vi "PoseAndTargeting.vi"() -> ()   [LabVIEW 2020]
doc: "Manages the robot's pose (position, heading, and velocity) and targeting information. Data from the IMU, swerve drive encoders, swerve azimuth encoders, turret enoder, and LimeLight are fused together to estimate these values. Supports pose resets on boot, from the Autonomous Sequencer, and on command from the FRC 4265 Dashboard."
uses:
  c71665c3-219d-469c-9b81-2f0818bb1921.vi
  sensordata.vi
  driverdata.vi
  robotoutputs.vi
panel:
  in  "Firing Delay (s)":dbl
  in  "Radial Target Shift (in)":dbl
  in  "Angular Target Shift (deg)":dbl
  in  "Min Timed Aligned (ms)":u32=500
  in  "Acceptable Heading Error (deg)":dbl=4.0
  in  "Vision Trust Threshold (in)":dbl=10.0
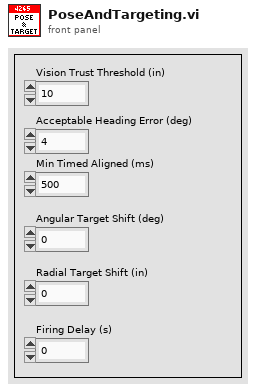
[diagram p1: front panel]
types:
  T1 = enum16{"Normal", "Auto Set", "Reset IMU", "Manual Push", "Init"}
  T2 = enum16{"Center", "North", "NorthWest", "West", "SouthWest", "South", "SouthEast", "East", "NorthEast"}
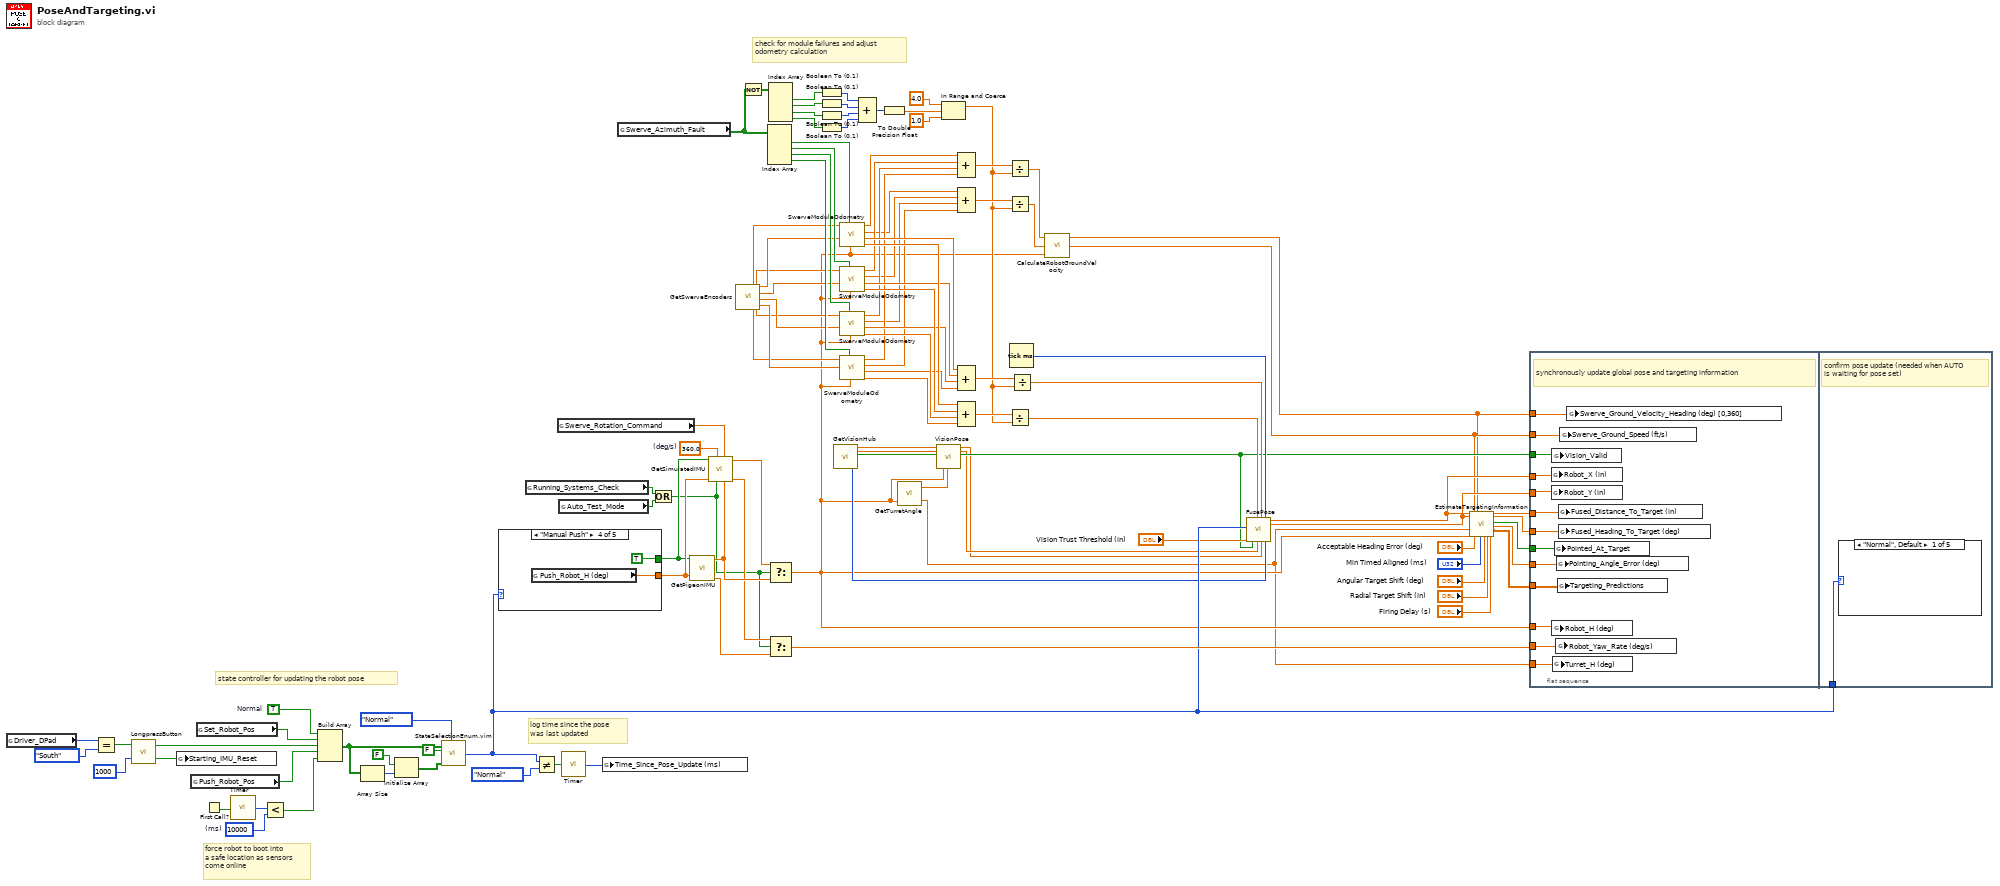
[diagram p0: block diagram]
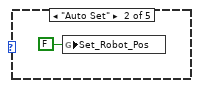
[diagram p2: hidden frame]
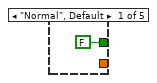
[diagram p6: hidden frame]
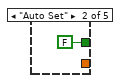
[diagram p7: hidden frame]
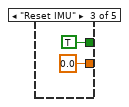
[diagram p8: hidden frame]
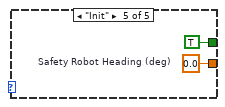
[diagram p9: hidden frame]
diagram:
  w79 = 360.0  # (deg/s)
  w83 = u32 10000  # (ms)
  w89 = TRUE  # Normal
  # "force robot to boot into\na safe location as sensors\ncome online"
  # "log time since the pose\nwas last updated"
  # "state controller for updating the robot pose"
  # "check for module failures and adjust\nodometry calculation"
  n1 = global read "driverdata.vi" "Driver_DPad"() -> (w46:T2)
  n2 = Equal?(x=w46, y=T2."South") -> (x = y?=w45:bool)
  n3 = call "LongpressButton.vi"("Threshold (ms)"=u32 1000, "Button"=w45) -> ("Starting Press"=w42:bool, "Longpress Button"=w43:bool)
  n4 = global write "driverdata.vi" "Starting_IMU_Reset"(w42) -> ()
  n5 = global read "sensordata.vi" "Push_Robot_Pos"() -> (w90:bool)
  n6 = global read "sensordata.vi" "Set_Robot_Pos"() -> (w78:bool)
  n7 = First Call?() -> (First Call?: T/F=w86:bool)
  n8 = call "Timer.vi"("Reset Timer"=w86) -> ("Time (ms)"=w85:u32)
  n9 = Less?(x=w85, y=w83) -> (x < y?=w84:bool)
  n10 = Build Array(w89, w78, w43, w90, w84) -> (w38:bool[])
  n11 = Array Size(array=w38) -> (size(s)=w41:i32)
  n12 = Initialize Array(FALSE, w41) -> (w37:bool[])
  n13 = call "StateSelectionEnum.vim"("Enum Def"=T1."Normal", "Disallowed States"=w37, "Enable Edge Trigger"=FALSE, "State Triggers"=w38) -> ("Selected State"=w28:T1)  [unwired: 1 in, 1 out]
  n14 = case shown="\"Manual Push\"" w28 {
    tunnel: [_ _ 0.0 ("Push_Robot_H (deg)") w118 w119] -> w82
    tunnel: [FALSE FALSE TRUE TRUE TRUE] -> w81
    frame "Normal", Default {
    }
    frame "Auto Set" {
    }
    frame "Reset IMU" {
    }
    frame "Manual Push" {
      n15 = global read "sensordata.vi" "Push_Robot_H (deg)"() -> (w118:dbl)
    }
    frame "Init" {
      w119 = 0.0  # Safety Robot Heading (deg)
    }
  }
  n16 = global read "driverdata.vi" "Running_Systems_Check"() -> (w33:bool)
  n17 = Not Equal?(x=w28, y=T1."Normal") -> (x != y?=w88:bool)
  n18 = global read "robotoutputs.vi" "Swerve_Rotation_Command"() -> (w80:dbl)
  n19 = global read "driverdata.vi" "Auto_Test_Mode"() -> (w34:bool)
  n20 = call "Timer.vi"("Reset Timer"=w88) -> ("Time (ms)"=w87:u32)
  n21 = global write "sensordata.vi" "Time_Since_Pose_Update (ms)"(w87) -> ()
  n22 = global read "sensordata.vi" "Swerve_Azimuth_Fault"() -> (w106:bool[])
  n23 = Or(x=w33, y=w34) -> (x .or. y?=w32:bool)
  n24 = call "GetPigeonIMU.vi"("Reset Yaw (deg)"=w82, "Reset Yaw"=w81) -> ("Yaw Rate (deg/s)"=w49:dbl, "Yaw (deg)"=w69:dbl)  [unwired: 6 in, 2 out]
  n25 = call "GetSimulatedIMU.vi"("Real IMU Yaw (deg)"=w69, "Rotation Command"=w80, "Auto Test Mode"=w32, "Max Simulated Rotation Speed (deg/s)"=w79, "Reset Yaw (deg)"=w82, "Reset Yaw"=w81) -> ("Simulated Yaw Rate (deg/s)"=w48:dbl, "Simulated Yaw (deg)"=w70:dbl)  [unwired: 2 in, 2 out]
  n26 = call "GetSwerveEncoders.vi"() -> ("Swerve 0 Velocity (ft/s)"=w53:dbl, "Swerve 3 Velocity (ft/s)"=w50:dbl, "Swerve 1 Velocity (ft/s)"=w52:dbl, "Swerve 2 Velocity (ft/s)"=w51:dbl, "Swerve 0 Azimuth Position (deg)"=w77:dbl, "Swerve 1 Azimuth Position (deg)"=w76:dbl, "Swerve 2 Azimuth Position (deg)"=w75:dbl, "Swerve 3 Azimuth Position (deg)"=w74:dbl)  [unwired: 20 in]
  n27 = Not(x=w106) -> (.not. x?=w105:bool[])
  n28 = Index Array(array=w106) -> (element #1=w95:bool, element #2=w94:bool, element #3=w93:bool, element #4=w92:bool)  [unwired: 4 in]
  n29 = Index Array(array=w105) -> (element #1=w104:bool, element #2=w103:bool, element #3=w102:bool, element #4=w101:bool)  [unwired: 4 in]
  n30 = Select(t=w70, s=w32, f=w69) -> (s? t:f=w9:dbl)
  n31 = Select(t=w48, s=w32, f=w49) -> (s? t:f=w47:dbl)
  n32 = Boolean To (0,1)(Boolean=w104) -> (0, 1=w100:i16)
  n33 = Boolean To (0,1)(Boolean=w103) -> (0, 1=w99:i16)
  n34 = Boolean To (0,1)(Boolean=w102) -> (0, 1=w98:i16)
  n35 = Boolean To (0,1)(Boolean=w101) -> (0, 1=w97:i16)
  n36 = call "GetVisionHub.vi"() -> ("Vision Timestamp (ms)"=w19:u32, "Vision Horizontal Angle to Target (deg) [t-?]"=w18:dbl, "Vision Vertical Angle to Target (deg) [t-?]"=w17:dbl, "Vision Target Valid [t-?]"=w16:bool)  [unwired: 16 in]
  n37 = call "SwerveModuleOdometry.vi"("Robot Heading(deg)"=w9, "Module Fault"=w95, "Wheel Azimuth (deg)"=w77, "Velocity (ft/s)"=w53) -> ("Delta Y (in)"=w107:dbl, "Delta X (in)"=w68:dbl, "Velocity Y (ft/s)"=w60:dbl, "Velocity X (ft/s)"=w64:dbl)  [unwired: 2 in]
  n38 = call "SwerveModuleOdometry.vi"("Robot Heading(deg)"=w9, "Module Fault"=w94, "Wheel Azimuth (deg)"=w76, "Velocity (ft/s)"=w52) -> ("Delta Y (in)"=w108:dbl, "Delta X (in)"=w67:dbl, "Velocity Y (ft/s)"=w59:dbl, "Velocity X (ft/s)"=w63:dbl)  [unwired: 2 in]
  n39 = call "SwerveModuleOdometry.vi"("Robot Heading(deg)"=w9, "Module Fault"=w93, "Wheel Azimuth (deg)"=w75, "Velocity (ft/s)"=w51) -> ("Delta Y (in)"=w109:dbl, "Delta X (in)"=w66:dbl, "Velocity Y (ft/s)"=w58:dbl, "Velocity X (ft/s)"=w62:dbl)  [unwired: 2 in]
  n40 = call "SwerveModuleOdometry.vi"("Robot Heading(deg)"=w9, "Module Fault"=w92, "Wheel Azimuth (deg)"=w74, "Velocity (ft/s)"=w50) -> ("Delta Y (in)"=w110:dbl, "Delta X (in)"=w65:dbl, "Velocity Y (ft/s)"=w57:dbl, "Velocity X (ft/s)"=w61:dbl)  [unwired: 2 in]
  n41 = Compound Arithmetic op=ADD(w100, w99, w98, w97) -> (w96:i16)
  n42 = To Double Precision Float(number=w96) -> (double precision float=w73:dbl)
  n43 = call "GetTurretAngle.vi"("Robot Heading (deg)"=w9) -> ("Turret Heading (deg)"=w8:dbl, "Turret Angle (deg)"=w10:dbl)  [unwired: 1 in]
  n44 = call "VisionPose.vi"("Vision Horizontal Angle to Target (deg) [t-?]"=w18, "Vision Vertical Angle to Target (deg) [t-?]"=w17, "Vision Target Valid [t-?]"=w16, "Robot Heading (deg)"=w9, "Turret Angle (deg)"=w10) -> ("Vision X (in) [t-?]"=w13:dbl, "Vision Y (in) [t-?]"=w14:dbl, "Vision Valid [t-?]"=w15:bool)  [unwired: 12 in]
  n45 = In Range and Coerce(upper limit=4.0, x=w73, lower limit=1.0) -> (coerced(x)=w54:dbl)  [unwired: 1 out]
  n46 = Compound Arithmetic op=ADD(w64, w63, w62, w61) -> (w56:dbl)
  n47 = Compound Arithmetic op=ADD(w60, w59, w58, w57) -> (w55:dbl)
  n48 = Compound Arithmetic op=ADD(w68, w67, w66, w65) -> (w112:dbl)
  n49 = Compound Arithmetic op=ADD(w107, w108, w109, w110) -> (w111:dbl)
  n50 = Divide(x=w56, y=w54) -> (x/y=w11:dbl)
  n51 = Divide(x=w55, y=w54) -> (x/y=w12:dbl)
  n52 = Divide(x=w111, y=w54) -> (x/y=w29:dbl)
  n53 = Tick Count (ms)() -> (millisecond timer value=w31:u32)
  n54 = Divide(x=w112, y=w54) -> (x/y=w30:dbl)
  n55 = call "CalculateRobotGroundVelocity.vi"("Robot Heading (deg)"=w9, "Velocity Y (ft/s)"=w12, "Velocity X (ft/s)"=w11) -> ("Velocity Magnitude (ft/s)"=w2:dbl, "Velocity Heading (deg)"=w1:dbl)  [unwired: 1 in]
  n56 = call "FusePose.vi"("Pose Mode"=w28, "Vision Trust Threshold (in)"="Vision Trust Threshold (in)", "Vision Valid [t-?]"=w15, "Odometry Delta Y (in) [t0]"=w29, "Vision Y (in) [t-?]"=w14, "Odometry Delta X (in) [t0]"=w30, "Vision X (in) [t-?]"=w13, "Odometry Timestamp (ms)"=w31, "Vision Timestamp (ms)"=w19) -> ("X (in) [t0]"=w23:dbl, "Y (in) [t0]"=w22:dbl)  [unwired: 9 in]
  n57 = call "EstimateTargetingInformation.vi"("X (in) [t0]"=w23, "Y (in) [t0]"=w22, "Turret Heading (deg)"=w8, "Robot Heading (deg)"=w9, "Velocity Magnitude (ft/s)"=w2, "Acceptable Heading Error (deg)"="Acceptable Heading Error (deg)", "Velocity Heading (deg)"=w1, "Min Timed Aligned (ms)"="Min Timed Aligned (ms)", "Angular Target Shift (deg)"="Angular Target Shift (deg)", "Radial Target Shift (in)"="Radial Target Shift (in)", "Firing Delay (s)"="Firing Delay (s)") -> ("Fused Distance to Target (in)"=w26:dbl, "Fused Heading to Target (deg)"=w25:dbl, "Pointed At Target"=w24:bool, "Pointing Angle Error (deg)"=w7:dbl, "Targeting Predictions"=w4:dbl[])  [unwired: 12 in]
  n58 = flat-sequence {
    tunnel: w9 -> [w133]
    tunnel: w47 -> [w132]
    tunnel: w26 -> [w131]
    tunnel: w25 -> [w130]
    tunnel: w24 -> [w129]
    tunnel: w23 -> [w128]
    tunnel: w22 -> [w127]
    tunnel: w15 -> [w126]
    tunnel: w8 -> [w125]
    tunnel: w7 -> [w124]
    tunnel: w2 -> [w123]
    tunnel: w1 -> [w122]
    tunnel: w4 -> [w121]
    tunnel: w28 -> [w134]
    frame #0 {
      # "synchronously update global pose and targeting information"
      n59 = global write "sensordata.vi" "Robot_X (in)"(w128) -> ()
      n60 = global write "sensordata.vi" "Robot_Y (in)"(w127) -> ()
      n61 = global write "sensordata.vi" "Vision_Valid"(w126) -> ()
      n62 = global write "sensordata.vi" "Robot_H (deg)"(w133) -> ()
      n63 = global write "sensordata.vi" "Turret_H (deg)"(w125) -> ()
      n64 = global write "sensordata.vi" "Pointed_At_Target"(w129) -> ()
      n65 = global write "sensordata.vi" "Robot_Yaw_Rate (deg/s)"(w132) -> ()
      n66 = global write "sensordata.vi" "Pointing_Angle_Error (deg)"(w124) -> ()
      n67 = global write "sensordata.vi" "Targeting_Predictions"(w121) -> ()
      n68 = global write "sensordata.vi" "Fused_Distance_To_Target (in)"(w131) -> ()
      n69 = global write "sensordata.vi" "Fused_Heading_To_Target (deg)"(w130) -> ()
      n70 = global write "sensordata.vi" "Swerve_Ground_Speed (ft/s)"(w123) -> ()
      n71 = global write "sensordata.vi" "Swerve_Ground_Velocity_Heading (deg) [0,360]"(w122) -> ()
    }
    frame #1 {
      # "confirm pose update (needed when AUTO is waiting for pose set)"
      n72 = case shown="\"Normal\", Default" w134 {
        frame "Normal", Default {
        }
        frame "Auto Set" {
          n73 = global write "sensordata.vi" "Set_Robot_Pos"(FALSE ("Set_Robot_Pos")) -> ()
        }
        frame "Reset IMU" {
        }
        frame "Manual Push" {
        }
        frame "Init" {
        }
      }
    }
  }
